vi "FetchAxisSharedVars.vi"(8 "error in (no error)":errorcluster caption="entrée d'erreur (pas d'erreur)", 9 "Numéro d'Axe":u32, 11 "PilMOT Address":string="ni.var.psp://localhost/OPC/OPC1/esbimETH_1") -> (0 "error out":errorcluster caption="sortie d'erreur", 1 "Sortie Variables d'Axes":T1)   [LabVIEW 2014]
doc: "Crée les chaînes de caractères permettant de lire et d'écrire les variables partagées du PilMOT. \nAV 18/11/2013"
uses:
  AdressesVariablesPartagees.ctl
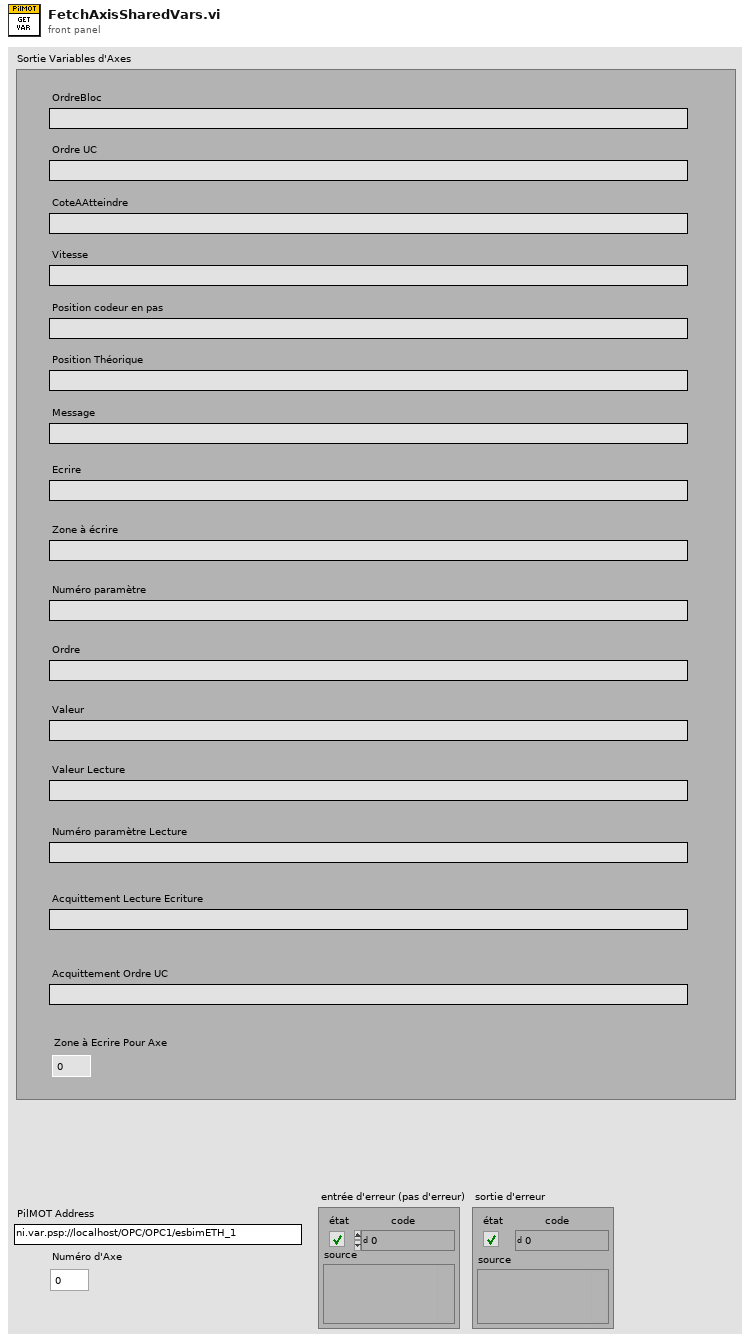
[diagram p1: front panel]
types:
  T1 = typedef "AdressesVariablesPartagees.ctl" = cluster{"OrdreBloc":string, "Ordre UC":string, "CoteAAtteindre":string, "Vitesse":string, "Position codeur en pas":string, "Position Théorique":string, "Message":string, "Ecrire":string, "Zone à écrire":string, "Numéro paramètre":string, "Ordre":string, "Valeur":string, "Valeur Lecture":string, "Numéro paramètre Lecture":string, "Acquittement Lecture Ecriture":string, "Zone à Ecrire Pour Axe ":u16, "Acquittement Ordre UC":string}
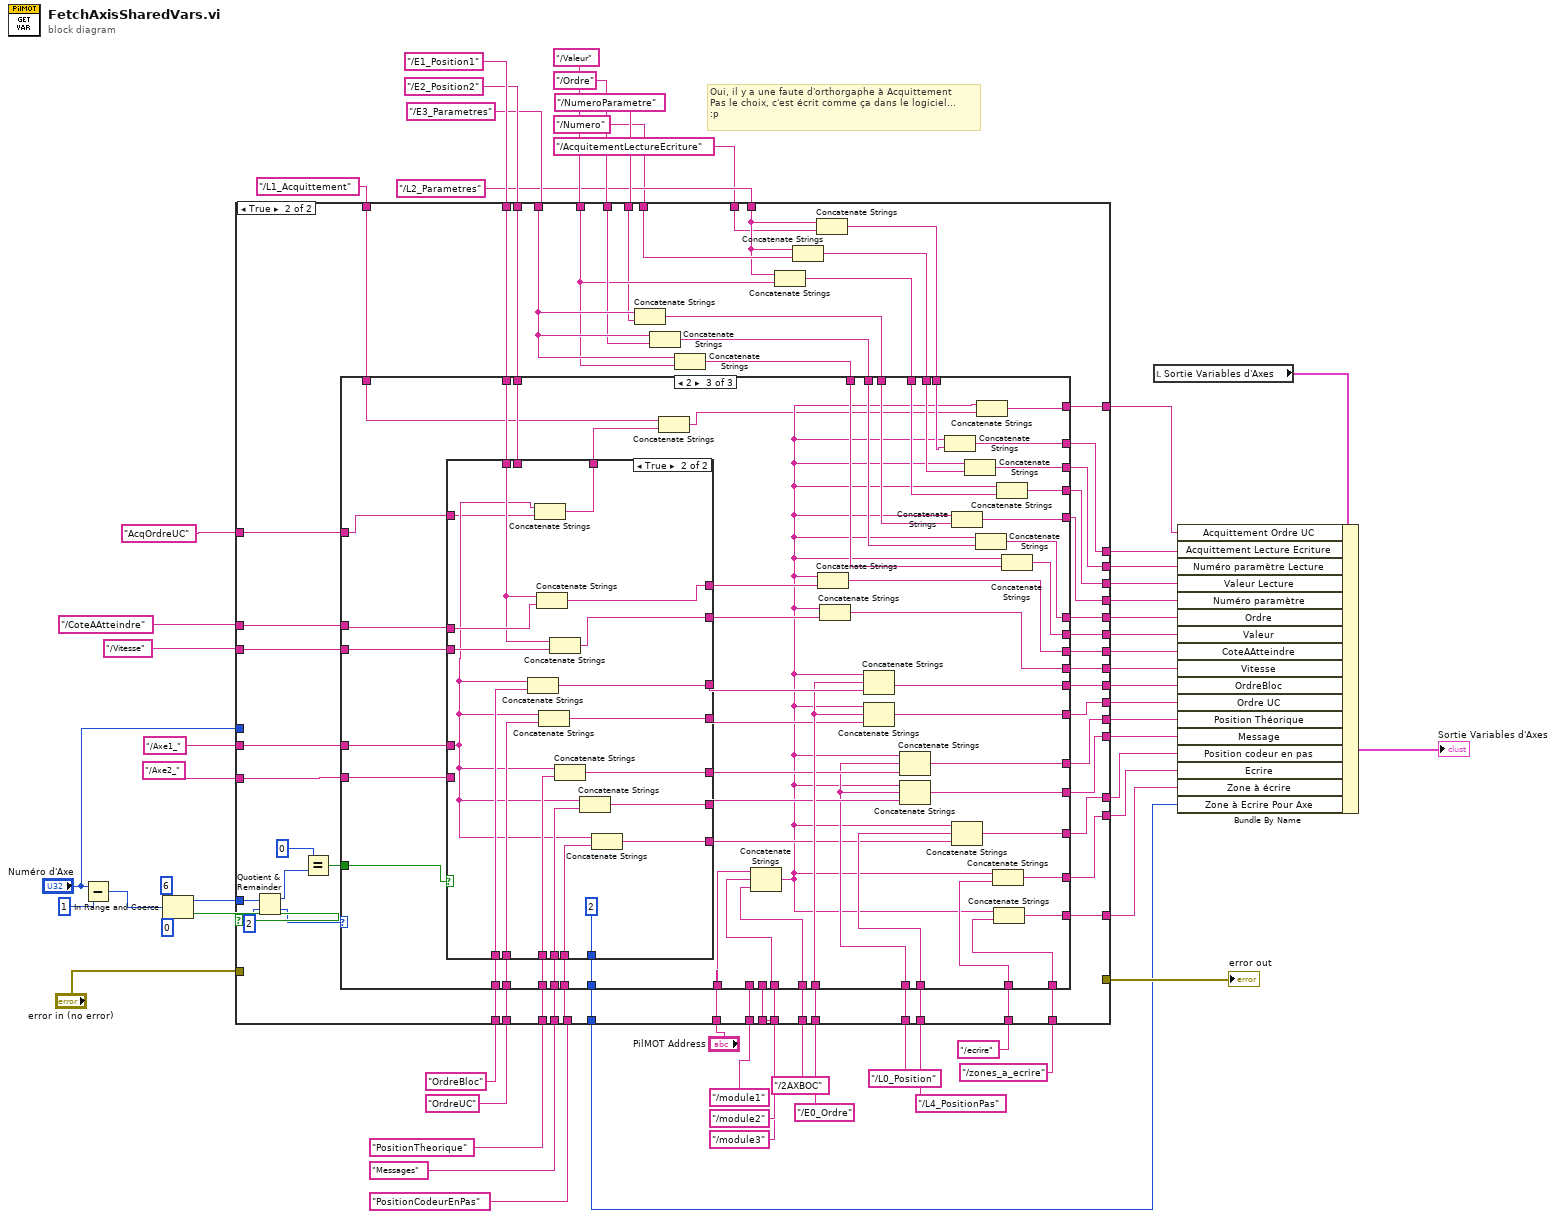
[diagram p0: block diagram]
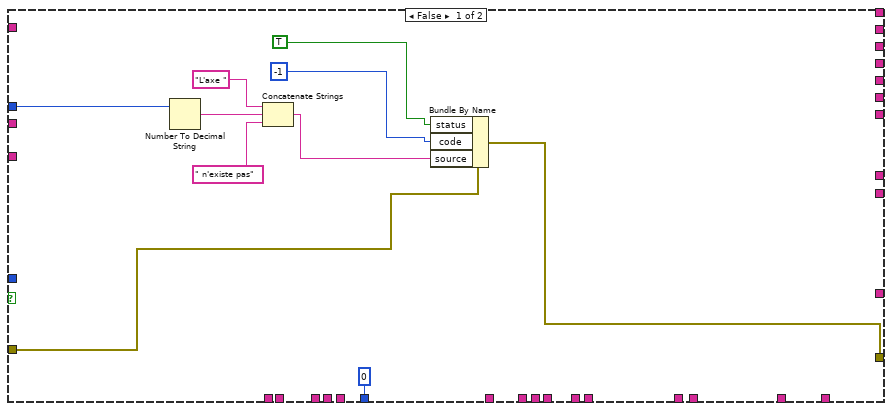
[diagram p2: hidden frame]
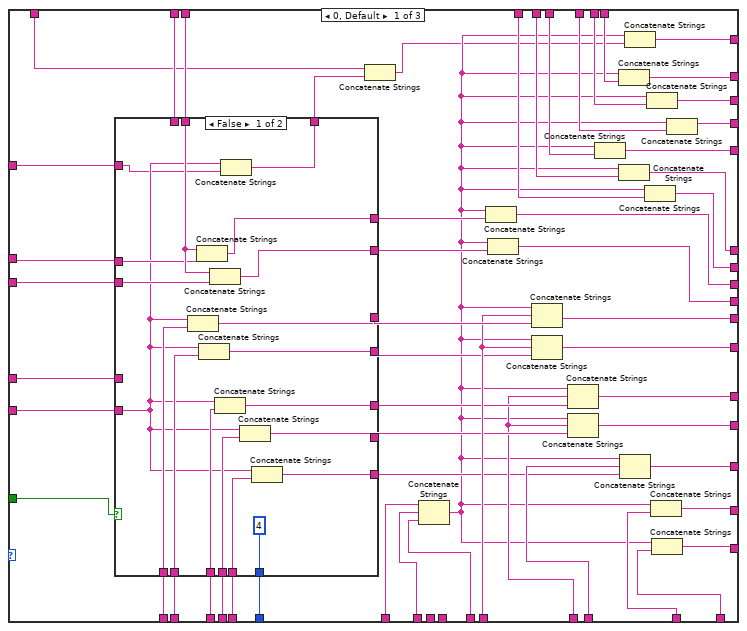
[diagram p3: hidden frame]
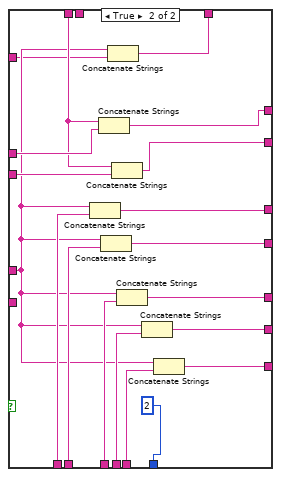
[diagram p4: hidden frame]
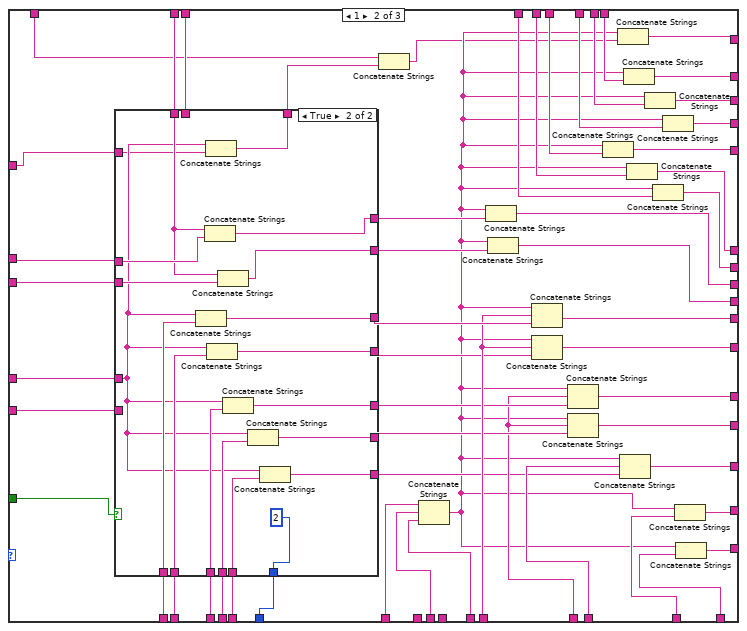
[diagram p5: hidden frame]
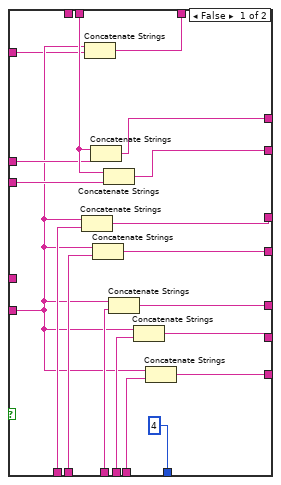
[diagram p6: hidden frame]
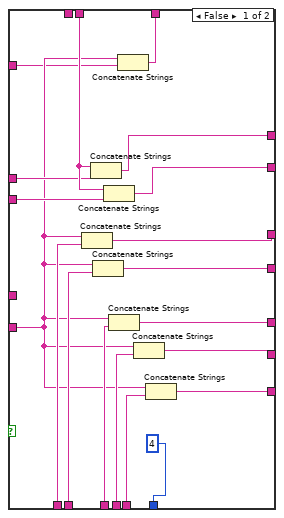
[diagram p7: hidden frame]
diagram:
  # "Oui, il y a une faute d'orthorgaphe à Acquittement\nPas le choix, c'est écrit comme ça dans le logiciel... \n:p"
  n1 = Subtract(x="Numéro d'Axe", y=u32 1) -> (x-y=w23:u32)
  n2 = In Range and Coerce(upper limit=u32 6 ("limite supérieure"), x=w23, lower limit=u32 0 ("y")) -> (coerced(x)=w55:u32, In Range?=w56:bool)
  n3 = case shown="True" w56 {
    tunnel: w55 -> [_ w97]
    tunnel: "error in (no error)" -> [w66 _]
    tunnel: [w65 _] -> w53
    tunnel: "/E1_Position1" -> [_ w122]
    tunnel: "/E2_Position2" -> [_ w121]
    tunnel: "/L0_Position" -> [_ w110]
    tunnel: "/L4_PositionPas" -> [_ w109]
    tunnel: "OrdreBloc" -> [_ w123]
    tunnel: "OrdreUC" -> [_ w120]
    tunnel: "PositionCodeurEnPas" -> [_ w117]
    tunnel: "Messages" -> [_ w118]
    tunnel: "PositionTheorique" -> [_ w119]
    tunnel: "/Axe1_" -> [_ w125]
    tunnel: "/Axe2_" -> [_ w124]
    tunnel: "PilMOT Address" -> [_ w127]
    tunnel: "/2AXBOC" -> [_ w126]
    tunnel: "/CoteAAtteindre" -> [_ w116]
    tunnel: "/Vitesse" -> [_ w115]
    tunnel: "/module1" -> [_ w114]
    tunnel: "/module2" -> [_ w113]
    tunnel: "/module3" -> [_ w112]
    tunnel: "/E0_Ordre" -> [_ w111]
    tunnel: [_ w108] -> w31
    tunnel: [_ w107] -> w30
    tunnel: [_ w106] -> w29
    tunnel: [_ w105] -> w28
    tunnel: [_ w104] -> w27
    tunnel: [_ w103] -> w26
    tunnel: [_ w102] -> w25
    tunnel: "Numéro d'Axe" -> [w60 _]
    tunnel: "/ecrire" -> [_ w95]
    tunnel: "/zones_a_ecrire" -> [_ w94]
    tunnel: [_ w93] -> w19
    tunnel: [_ w92] -> w18
    tunnel: "/E3_Parametres" -> [_ w91]
    tunnel: "/Valeur" -> [_ w83]
    tunnel: "/Ordre" -> [_ w90]
    tunnel: "/NumeroParametre" -> [_ w82]
    tunnel: [_ w86] -> w13
    tunnel: [_ w85] -> w12
    tunnel: [_ w84] -> w11
    tunnel: "/L2_Parametres" -> [_ w76]
    tunnel: [_ w80] -> w9
    tunnel: "/Numero" -> [_ w79]
    tunnel: [_ w77] -> w7
    tunnel: "/AcquitementLectureEcriture" -> [_ w75]
    tunnel: [_ w73] -> w5
    tunnel: [u16 0 w72] -> w4
    tunnel: "AcqOrdreUC" -> [_ w71]
    tunnel: "/L1_Acquittement" -> [_ w70]
    tunnel: [_ w69] -> w1
    frame False {
      n4 = Number To Decimal String(number=w60) -> (decimal integer string=w61:string)  [unwired: 1 in]
      n5 = Concatenate Strings("L'axe " ("chaîne"), w61, " n'existe pas" ("chaîne")) -> (w62:string)
      n6 = Bundle By Name(cluster=w66, "status"=TRUE, "code"=-1, "source"=w62) -> (w65:errorcluster)
    }
    frame True {
      n7 = Quotient & Remainder(x=w97, y=u32 2) -> (x-y*floor(x/y)=w100:u32, floor(x/y)=w96:u32)
      n8 = Equal?(x=u32 0, y=w100) -> (x = y?=w98:bool)
      n9 = Concatenate Strings(w91, w82) -> (w87:string)
      n10 = Concatenate Strings(w91, w90) -> (w88:string)
      n11 = Concatenate Strings(w91, w83) -> (w89:string)
      n12 = Concatenate Strings(w76, w83) -> (w81:string)
      n13 = Concatenate Strings(w76, w79) -> (w78:string)
      n14 = Concatenate Strings(w76, w75) -> (w74:string)
      n15 = case shown="2" w96 {
        tunnel: w127 -> [w171 w264 w357]
        tunnel: w126 -> [w169 w263 w356]
        tunnel: w125 -> [w172 w265 w358]
        tunnel: w124 -> [w182 w275 w368]
        tunnel: w123 -> [w181 w274 w367]
        tunnel: w122 -> [w180 w273 w366]
        tunnel: w121 -> [w179 w272 w365]
        tunnel: w120 -> [w178 w271 w364]
        tunnel: w119 -> [w177 w270 w363]
        tunnel: w118 -> [w176 w269 w362]
        tunnel: w117 -> [w175 w268 w361]
        tunnel: w116 -> [w174 w267 w360]
        tunnel: w115 -> [w173 w266 w359]
        tunnel: w114 -> [w170 _ _]
        tunnel: w113 -> [_ w244 _]
        tunnel: w112 -> [_ _ w337]
        tunnel: w111 -> [w165 w259 w352]
        tunnel: w110 -> [w161 w255 w348]
        tunnel: w109 -> [w160 w254 w347]
        tunnel: [w158 w252 w345] -> w108
        tunnel: [w157 w251 w344] -> w107
        tunnel: [w156 w250 w343] -> w106
        tunnel: [w155 w249 w342] -> w105
        tunnel: [w154 w248 w341] -> w104
        tunnel: [w153 w247 w340] -> w103
        tunnel: [w152 w246 w339] -> w102
        tunnel: w98 -> [w151 w245 w338]
        tunnel: w95 -> [w150 w243 w336]
        tunnel: w94 -> [w149 w242 w335]
        tunnel: [w147 w241 w334] -> w93
        tunnel: [w148 w240 w333] -> w92
        tunnel: w89 -> [w146 w239 w332]
        tunnel: w88 -> [w145 w238 w331]
        tunnel: w87 -> [w144 w237 w330]
        tunnel: [w143 w236 w329] -> w86
        tunnel: [w142 w235 w328] -> w85
        tunnel: [w141 w234 w327] -> w84
        tunnel: w81 -> [w140 w233 w326]
        tunnel: [w139 w232 w325] -> w80
        tunnel: w78 -> [w138 w231 w324]
        tunnel: [w137 w230 w323] -> w77
        tunnel: w74 -> [w136 w229 w322]
        tunnel: [w135 w228 w321] -> w73
        tunnel: [w134 w227 w320] -> w72
        tunnel: w71 -> [w133 w226 w319]
        tunnel: w70 -> [w130 w224 w317]
        tunnel: [w128 w221 w314] -> w69
        frame 0, Default {
          n16 = case shown="False" w151 {
            tunnel: w182 -> [w185 _]
            tunnel: w181 -> [w201 w217]
            tunnel: w180 -> [_ w218]
            tunnel: w179 -> [w196 _]
            tunnel: w178 -> [w200 w216]
            tunnel: w177 -> [w199 w215]
            tunnel: w176 -> [w198 w214]
            tunnel: w175 -> [w197 w213]
            tunnel: w174 -> [w194 w220]
            tunnel: w173 -> [w195 w219]
            tunnel: w172 -> [_ w204]
            tunnel: [w193 w212] -> w168
            tunnel: [w192 w206] -> w167
            tunnel: [w191 w211] -> w166
            tunnel: [w190 w210] -> w164
            tunnel: [w189 w209] -> w163
            tunnel: [w188 w208] -> w162
            tunnel: [w187 w207] -> w159
            tunnel: [u16 4 u16 2] -> w134
            tunnel: w133 -> [w184 w203]
            tunnel: [w183 w202] -> w131
            frame False {
              n17 = Concatenate Strings(w185, w201) -> (w191:string)
              n18 = Concatenate Strings(w196, w194) -> (w193:string)
              n19 = Concatenate Strings(w185, w200) -> (w190:string)
              n20 = Concatenate Strings(w196, w195) -> (w192:string)
              n21 = Concatenate Strings(w185, w199) -> (w189:string)
              n22 = Concatenate Strings(w185, w184) -> (w183:string)
              n23 = Concatenate Strings(w185, w198) -> (w188:string)
              n24 = Concatenate Strings(w185, w197) -> (w187:string)
            }
            frame True {
              n25 = Concatenate Strings(w204, w217) -> (w211:string)
              n26 = Concatenate Strings(w218, w220) -> (w212:string)
              n27 = Concatenate Strings(w204, w216) -> (w210:string)
              n28 = Concatenate Strings(w204, w203) -> (w202:string)
              n29 = Concatenate Strings(w218, w219) -> (w206:string)
              n30 = Concatenate Strings(w204, w215) -> (w209:string)
              n31 = Concatenate Strings(w204, w214) -> (w208:string)
              n32 = Concatenate Strings(w204, w213) -> (w207:string)
            }
          }
          n33 = Concatenate Strings(w130, w131) -> (w129:string)
          n34 = Concatenate Strings(w171, w170, w169) -> (w132:string)
          n35 = Concatenate Strings(w132, w168) -> (w158:string)
          n36 = Concatenate Strings(w132, w167) -> (w157:string)
          n37 = Concatenate Strings(w132, w165, w166) -> (w156:string)
          n38 = Concatenate Strings(w132, w165, w164) -> (w155:string)
          n39 = Concatenate Strings(w132, w161, w163) -> (w154:string)
          n40 = Concatenate Strings(w132, w161, w162) -> (w153:string)
          n41 = Concatenate Strings(w132, w144) -> (w143:string)
          n42 = Concatenate Strings(w132, w136) -> (w135:string)
          n43 = Concatenate Strings(w132, w145) -> (w142:string)
          n44 = Concatenate Strings(w132, w160, w159) -> (w152:string)
          n45 = Concatenate Strings(w132, w129) -> (w128:string)
          n46 = Concatenate Strings(w132, w146) -> (w141:string)
          n47 = Concatenate Strings(w132, w138) -> (w137:string)
          n48 = Concatenate Strings(w132, w150) -> (w147:string)
          n49 = Concatenate Strings(w132, w149) -> (w148:string)
          n50 = Concatenate Strings(w132, w140) -> (w139:string)
        }
        frame 1 {
          n51 = case shown="True" w245 {
            tunnel: w275 -> [w278 _]
            tunnel: w274 -> [w294 w310]
            tunnel: w273 -> [_ w311]
            tunnel: w272 -> [w289 _]
            tunnel: w271 -> [w293 w309]
            tunnel: w270 -> [w292 w308]
            tunnel: w269 -> [w291 w307]
            tunnel: w268 -> [w290 w306]
            tunnel: w267 -> [w287 w313]
            tunnel: w266 -> [w288 w312]
            tunnel: w265 -> [_ w297]
            tunnel: [w286 w305] -> w262
            tunnel: [w285 w299] -> w261
            tunnel: [w284 w304] -> w260
            tunnel: [w283 w303] -> w258
            tunnel: [w282 w302] -> w257
            tunnel: [w281 w301] -> w256
            tunnel: [w280 w300] -> w253
            tunnel: [u16 4 u16 2] -> w227
            tunnel: w226 -> [w277 w296]
            tunnel: [w276 w295] -> w225
            frame False {
              n52 = Concatenate Strings(w278, w294) -> (w284:string)
              n53 = Concatenate Strings(w278, w277) -> (w276:string)
              n54 = Concatenate Strings(w289, w287) -> (w286:string)
              n55 = Concatenate Strings(w278, w293) -> (w283:string)
              n56 = Concatenate Strings(w289, w288) -> (w285:string)
              n57 = Concatenate Strings(w278, w292) -> (w282:string)
              n58 = Concatenate Strings(w278, w291) -> (w281:string)
              n59 = Concatenate Strings(w278, w290) -> (w280:string)
            }
            frame True {
              n60 = Concatenate Strings(w297, w310) -> (w304:string)
              n61 = Concatenate Strings(w311, w313) -> (w305:string)
              n62 = Concatenate Strings(w297, w296) -> (w295:string)
              n63 = Concatenate Strings(w297, w309) -> (w303:string)
              n64 = Concatenate Strings(w311, w312) -> (w299:string)
              n65 = Concatenate Strings(w297, w308) -> (w302:string)
              n66 = Concatenate Strings(w297, w307) -> (w301:string)
              n67 = Concatenate Strings(w297, w306) -> (w300:string)
            }
          }
          n68 = Concatenate Strings(w224, w225) -> (w222:string)
          n69 = Concatenate Strings(w264, w244, w263) -> (w223:string)
          n70 = Concatenate Strings(w223, w262) -> (w252:string)
          n71 = Concatenate Strings(w223, w261) -> (w251:string)
          n72 = Concatenate Strings(w223, w259, w260) -> (w250:string)
          n73 = Concatenate Strings(w223, w259, w258) -> (w249:string)
          n74 = Concatenate Strings(w223, w255, w257) -> (w248:string)
          n75 = Concatenate Strings(w223, w255, w256) -> (w247:string)
          n76 = Concatenate Strings(w223, w237) -> (w236:string)
          n77 = Concatenate Strings(w223, w222) -> (w221:string)
          n78 = Concatenate Strings(w223, w254, w253) -> (w246:string)
          n79 = Concatenate Strings(w223, w229) -> (w228:string)
          n80 = Concatenate Strings(w223, w238) -> (w235:string)
          n81 = Concatenate Strings(w223, w231) -> (w230:string)
          n82 = Concatenate Strings(w223, w239) -> (w234:string)
          n83 = Concatenate Strings(w223, w233) -> (w232:string)
          n84 = Concatenate Strings(w223, w243) -> (w241:string)
          n85 = Concatenate Strings(w223, w242) -> (w240:string)
        }
        frame 2 {
          n86 = case shown="True" w338 {
            tunnel: w368 -> [w371 _]
            tunnel: w367 -> [w387 w403]
            tunnel: w366 -> [_ w404]
            tunnel: w365 -> [w382 _]
            tunnel: w364 -> [w386 w402]
            tunnel: w363 -> [w385 w401]
            tunnel: w362 -> [w384 w400]
            tunnel: w361 -> [w383 w399]
            tunnel: w360 -> [w380 w406]
            tunnel: w359 -> [w381 w405]
            tunnel: w358 -> [_ w390]
            tunnel: [w379 w398] -> w355
            tunnel: [w378 w392] -> w354
            tunnel: [w377 w397] -> w353
            tunnel: [w376 w396] -> w351
            tunnel: [w375 w395] -> w350
            tunnel: [w374 w394] -> w349
            tunnel: [w373 w393] -> w346
            tunnel: [u16 4 u16 2] -> w320
            tunnel: w319 -> [w370 w389]
            tunnel: [w369 w388] -> w318
            frame False {
              n87 = Concatenate Strings(w371, w387) -> (w377:string)
              n88 = Concatenate Strings(w382, w380) -> (w379:string)
              n89 = Concatenate Strings(w371, w386) -> (w376:string)
              n90 = Concatenate Strings(w382, w381) -> (w378:string)
              n91 = Concatenate Strings(w371, w385) -> (w375:string)
              n92 = Concatenate Strings(w371, w370) -> (w369:string)
              n93 = Concatenate Strings(w371, w384) -> (w374:string)
              n94 = Concatenate Strings(w371, w383) -> (w373:string)
            }
            frame True {
              n95 = Concatenate Strings(w390, w403) -> (w397:string)
              n96 = Concatenate Strings(w390, w389) -> (w388:string)
              n97 = Concatenate Strings(w404, w406) -> (w398:string)
              n98 = Concatenate Strings(w390, w402) -> (w396:string)
              n99 = Concatenate Strings(w404, w405) -> (w392:string)
              n100 = Concatenate Strings(w390, w401) -> (w395:string)
              n101 = Concatenate Strings(w390, w400) -> (w394:string)
              n102 = Concatenate Strings(w390, w399) -> (w393:string)
            }
          }
          n103 = Concatenate Strings(w317, w318) -> (w315:string)
          n104 = Concatenate Strings(w357, w337, w356) -> (w316:string)
          n105 = Concatenate Strings(w316, w355) -> (w345:string)
          n106 = Concatenate Strings(w316, w354) -> (w344:string)
          n107 = Concatenate Strings(w316, w352, w353) -> (w343:string)
          n108 = Concatenate Strings(w316, w352, w351) -> (w342:string)
          n109 = Concatenate Strings(w316, w348, w350) -> (w341:string)
          n110 = Concatenate Strings(w316, w348, w349) -> (w340:string)
          n111 = Concatenate Strings(w316, w322) -> (w321:string)
          n112 = Concatenate Strings(w316, w330) -> (w329:string)
          n113 = Concatenate Strings(w316, w347, w346) -> (w339:string)
          n114 = Concatenate Strings(w316, w324) -> (w323:string)
          n115 = Concatenate Strings(w316, w331) -> (w328:string)
          n116 = Concatenate Strings(w316, w315) -> (w314:string)
          n117 = Concatenate Strings(w316, w336) -> (w334:string)
          n118 = Concatenate Strings(w316, w335) -> (w333:string)
          n119 = Concatenate Strings(w316, w326) -> (w325:string)
          n120 = Concatenate Strings(w316, w332) -> (w327:string)
        }
      }
    }
  }
  "error out" <- w53
  n121 = local read "Sortie Variables d'Axes"() -> (w43:T1)
  n122 = Bundle By Name(cluster=w43, "Acquittement Ordre UC"=w1, "Acquittement Lecture Ecriture"=w5, "Numéro paramètre Lecture"=w7, "Valeur Lecture"=w9, "Numéro paramètre"=w13, "Ordre"=w12, "Valeur"=w11, "CoteAAtteindre"=w31, "Vitesse"=w30, "OrdreBloc"=w29, "Ordre UC"=w28, "Position Théorique"=w27, "Message"=w26, "Position codeur en pas"=w25, "Ecrire"=w19, "Zone à écrire"=w18, "Zone à Ecrire Pour Axe"=w4) -> (→"Sortie Variables d'Axes":T1)
